vi "ENA_E5072A.vi"() -> ()   [LabVIEW 2020]
uses:
  484af209-f5fb-4e97-a5fb-2c0625b22b84.vi
  <instrlib>/Agilent ENA Series/Agilent ENA Series.lvlib
panel:
  out "종료(숨김)":bool
  out "진행상황":string
  out "저장 카운터(숨김)":i32
  out "flag(숨김)":bool
  out "진행시간":string="0d 0h 0m 0s"
  in  "자동저장":bool
  in  "작동시간(분)":i32=120 min=1
  in  "주기(분)":i32=20 min=1
  out "최종저장횟수(숨김)":string
  out "종료시간":timestamp format="%<%X\n%x>T"
  out "시작(숨김)":timestamp format="%<%X\n%x>T"
  out "실수값 [dB]":dbl
  out "주파수 [MHz]":dbl
  out "Data sheet":string[][](table)
  in  "s2p 저장":bool caption="빈 버튼"
  in  "s2p 파일명":string caption="파일명"
  in  "파일명":string
  in  "저장경로":path
  in  "이미지 저장":bool caption="빈 버튼"
  in  "Reset":bool
  in  "라디오 버튼":enum32{"Center / Span", "Start / Stop"}(radio)
  in  "Stop [MHz]":dbl
  in  "Start [MHz]":dbl
  in  "Span [MHz]":dbl=2000.0
  in  "Center [MHz]":dbl=5000.0
  in  "Value Graticule Line (0.0)":dbl format="%^.2e"
  in  "Data Format":u16(ring) items=["Logarithmic Magnitude", "Phase", "Group Delay", "Smith Chart  Linear (Lin/Phase)", "Smith Chart  Logarithmic (Log/Phase)", "Smith Chart  Complex (Real/Imag)", "Smith Chart  Impedance (R+jX)", "Smith Chart  Admittance (G+jB)", "Polar Format (Linear)", "Polar Format (Logarithmic)", "Polar Format (Re/Im)", "Linear Magnitude", "SWR", "Real", "Imaginary", "Epanded Phase", "Positive Phase"]
  in  "Measurement Parameters":u16(ring)=1 items=["S11"=0, "S21"=1, "S12"=4, "S22"=5, "A"=16, "B"=17, "R1"=20, "R2"=21, "AUX1"=24, "AUX2"=25]
  in  "VISA Resource Name":refnum<visa-resource-name>
  in  "Hold":bool=TRUE
  out "Graph":cluster{"X":dbl, "Y":dbl}[](graph)
  in  "종료":bool
  in  "데이터 읽기":bool
  in  "설정":bool
  # "PEAK"
  # ".png"
  # ".s2p"
  # "by yys"
  # "Cont"
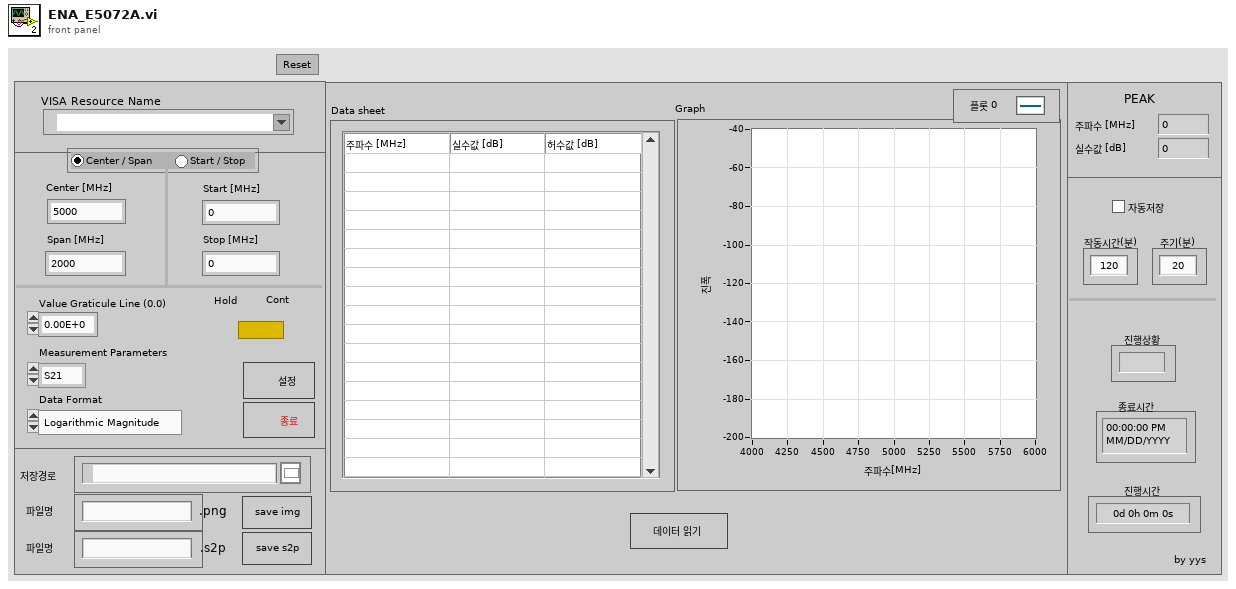
[diagram p1: front panel]
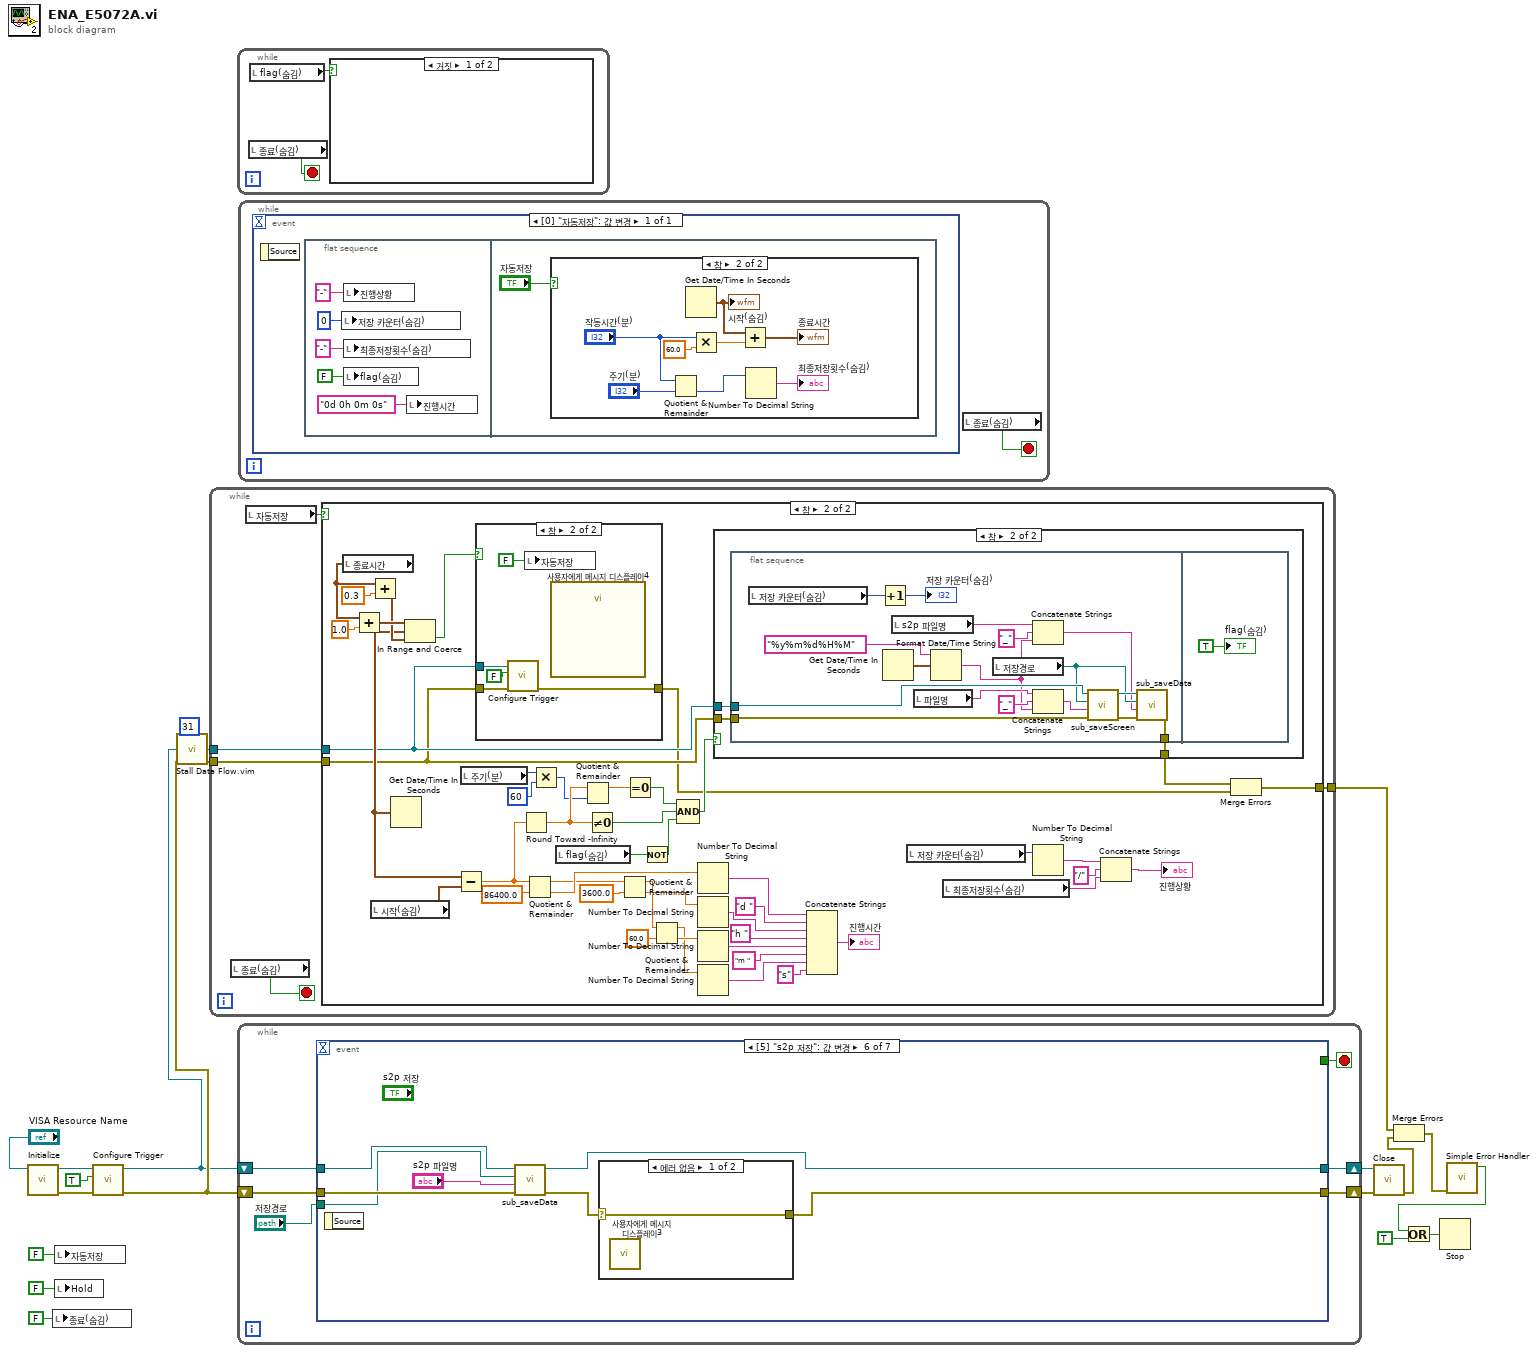
[diagram p0: block diagram]
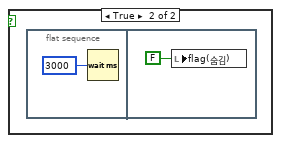
[diagram p5: hidden frame]
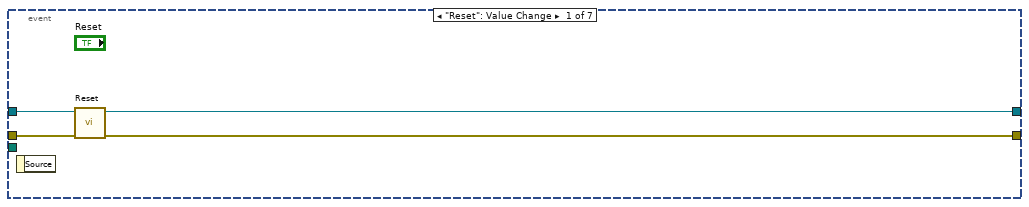
[diagram p7: hidden frame]
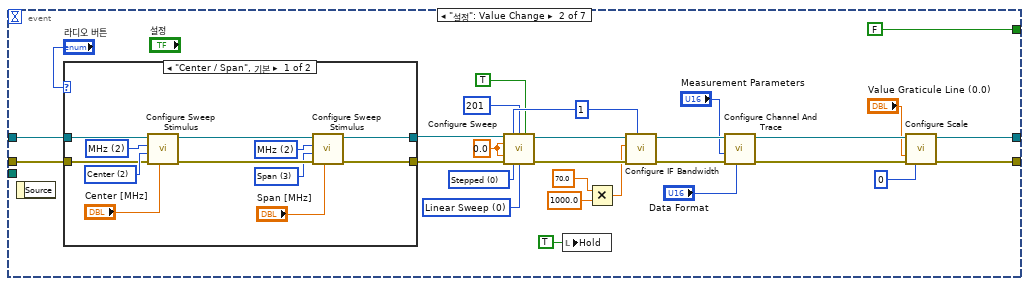
[diagram p8: hidden frame]
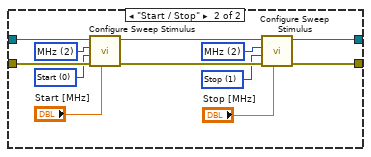
[diagram p9: hidden frame]
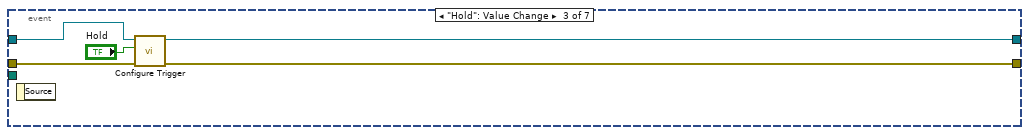
[diagram p10: hidden frame]
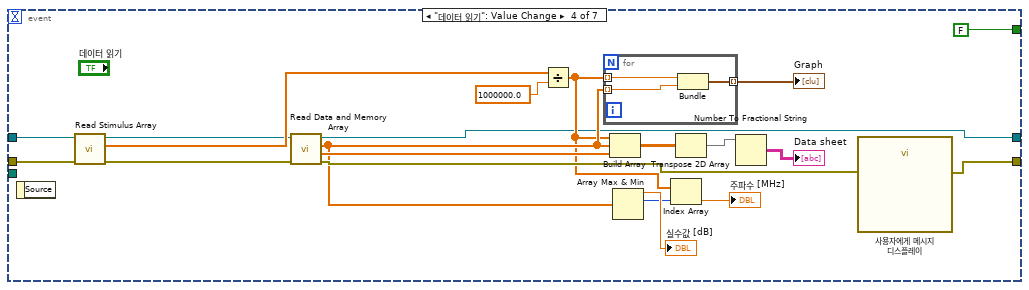
[diagram p11: hidden frame]
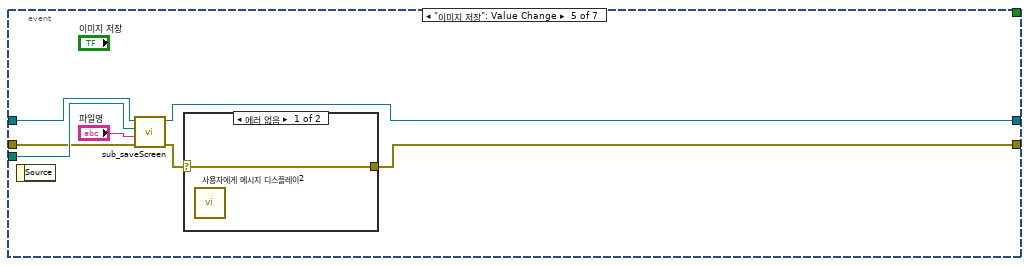
[diagram p12: hidden frame]
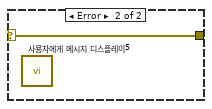
[diagram p13: hidden frame]
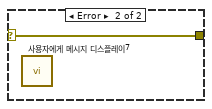
[diagram p14: hidden frame]
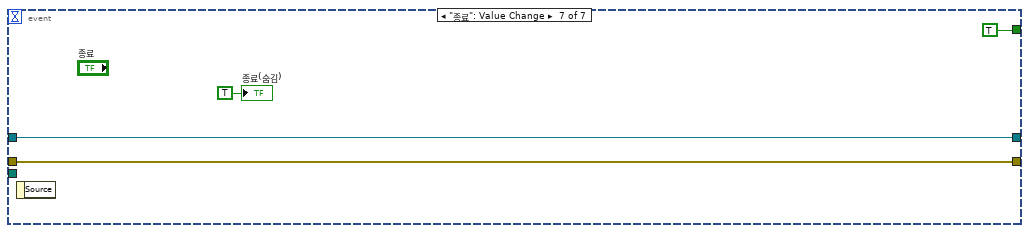
[diagram p15: hidden frame]
diagram:
  n1 = call <instrlib>:"Initialize.vi"("VISA resource name"="VISA Resource Name") -> ("error out"=w17:errorcluster, "VISA resource name out"=w18:refnum<visa-resource-name>)  [unwired: 9 in]
  n2 = local write "종료(숨김)"(FALSE ("종료(숨김)")) -> ()
  n3 = local write "자동저장"(FALSE ("자동저장")) -> ()
  n4 = local write "Hold"(FALSE ("Hold")) -> ()
  n5 = call <instrlib>:"Configure Trigger.vi"("error in (no error)"=w17, "Continuous Sweep (T: Enable)"=TRUE, "VISA resource name"=w18) -> ("error out"=w10:errorcluster, "VISA resource name out"=w9:refnum<visa-resource-name>)  [unwired: 7 in]
  n6 = call "Stall Data Flow.vim"("value in"=w9, "milliseconds to wait"=u32 31) -> ("value out"=w12:refnum<visa-resource-name>)  [unwired: 1 out]
  n7 = while {
    tunnel: w12 -> [w22]
    tunnel: w10 -> [w21]
    tunnel: [w20] -> w8
    stop <- w23 stop-if-true
    n8 = local read "종료(숨김)"() -> (w23:bool)
    n9 = local read "자동저장"() -> (w24:bool)
    n10 = case shown="참" w24 {
      tunnel: w22 -> [_ w30]
      tunnel: w21 -> [w25 w29]
      tunnel: [w25 w26] -> w20
      frame False {
      }
      frame True {
        n11 = local read "종료시간"() -> (w35:timestamp)
        n12 = Add(x=w35, y=1.0) -> (x+y=w42:timestamp)
        n13 = Add(x=w35, y=0.3) -> (x+y=w34:timestamp)
        n14 = local read "시작(숨김)"() -> (w53:timestamp)
        n15 = Get Date/Time In Seconds() -> (seconds since 1Jan1904=w31:timestamp)
        n16 = In Range and Coerce(upper limit=w42, x=w31, lower limit=w34) -> (In Range?=w44:bool)  [unwired: 1 out]
        n17 = Subtract(x=w31, y=w53) -> (x-y=w52:dbl)
        n18 = local read "주기(분)"() -> (w56:i32)
        n19 = case shown="참" w44 {
          tunnel: w30 -> [_ w76]
          tunnel: w29 -> [w73 w75]
          tunnel: [w73 w74] -> w28
          frame False {
          }
          frame True {
            n20 = call <instrlib>:"Configure Trigger.vi"("error in (no error)"=w75, "Continuous Sweep (T: Enable)"=FALSE, "VISA resource name"=w76) -> ("error out"=w74:errorcluster)  [unwired: 7 in, 1 out]
            n21 = local write "자동저장"(FALSE ("자동저장")) -> ()
            n22 = call "사용자에게 메시지 디스플레이4"() -> ()  [unwired: 10 in, 2 out]
          }
        }
        n23 = Round Toward -Infinity(1:w52) -> (0:w49:dbl)
        n24 = Quotient & Remainder(x=w52, y=86400.0) -> (x-y*floor(x/y)=w70:dbl, floor(x/y)=w72:dbl)
        n25 = Multiply(x=w56, y=60) -> (x*y=w45:i32)
        n26 = local read "flag(숨김)"() -> (w47:bool)
        n27 = Quotient & Remainder(x=w49, y=w45) -> (x-y*floor(x/y)=w54:dbl)  [unwired: 1 out]
        n28 = Not Equal To 0?(x=w49) -> (x != 0?=w50:bool)
        n29 = Quotient & Remainder(x=w70, y=3600.0) -> (x-y*floor(x/y)=w68:dbl, floor(x/y)=w71:dbl)
        n30 = Equal To 0?(x=w54) -> (x = 0?=w51:bool)
        n31 = Not(x=w47) -> (.not. x?=w46:bool)
        n32 = Quotient & Remainder(x=w68, y=60.0) -> (x-y*floor(x/y)=w67:dbl, floor(x/y)=w69:dbl)
        n33 = Compound Arithmetic op=AND ("복합 연산")(w51, w50, w46) -> (w48:bool)
        n34 = Number To Decimal String(number=w72) -> (decimal integer string=w32:string)  [unwired: 1 in]
        n35 = Number To Decimal String(number=w71) -> (decimal integer string=w66:string)  [unwired: 1 in]
        n36 = Number To Decimal String(number=w69) -> (decimal integer string=w65:string)  [unwired: 1 in]
        n37 = Number To Decimal String(number=w67) -> (decimal integer string=w64:string)  [unwired: 1 in]
        n38 = case shown="참" w48 {
          tunnel: w30 -> [_ w82]
          tunnel: w29 -> [w79 w81]
          tunnel: [w79 w80] -> w27
          frame False {
          }
          frame True {
            n39 = flat-sequence {
              tunnel: w82 -> [w98]
              tunnel: w81 -> [w86]
              tunnel: [w83] -> w80
              frame #0 {
                n40 = local read "저장 카운터(숨김)"() -> (w84:i32)
                n41 = Increment(x=w84) -> (x+1=→"저장 카운터(숨김)":i32)
                n42 = Get Date/Time In Seconds() -> (seconds since 1Jan1904=w95:timestamp)
                n43 = local read "s2p 파일명"() -> (w92:string)
                n44 = local read "파일명"() -> (w89:string)
                n45 = Format Date/Time String(time format string (%c)="%y%m%d%H%M" ("시간 포맷 문자열 (%c)"), seconds (now)=w95) -> (date/time string=w88:string)  [unwired: 1 in]
                n46 = local read "저장경로"() -> (w96:path)
                n47 = Concatenate Strings(w92, "_" ("문자열"), w88) -> (w91:string)
                n48 = Concatenate Strings(w89, "_" ("문자열"), w88) -> (w87:string)
                n49 = call "sub_saveScreen.vi"("에러 입력(에러 없음)"=w86, "파일명"=w87, "저장경로"=w96, "VISA 참조 번호 입력"=w98) -> ("에러 출력"=w85:errorcluster, "VISA 참조 번호 출력"=w97:refnum<visa-resource-name>)  [unwired: 6 in]
                n50 = call "sub_saveData.vi"("에러 입력(에러 없음)"=w85, "파일명"=w91, "저장경로"=w96, "VISA 참조 번호 입력"=w97) -> ("에러 출력"=w83:errorcluster)  [unwired: 6 in, 1 out]
              }
              frame #1 {
                "flag(숨김)" <- TRUE
              }
            }
          }
        }
        n51 = Concatenate Strings(w32, "d " ("문자열"), w66, "h " ("문자열"), w65, "m " ("문자열"), w64, "s" ("문자열")) -> (→"진행시간":string)
        n52 = local read "저장 카운터(숨김)"() -> (w39:i32)
        n53 = local read "최종저장횟수(숨김)"() -> (w33:string)
        n54 = Number To Decimal String(number=w39) -> (decimal integer string=w38:string)  [unwired: 1 in]
        n55 = Concatenate Strings(w38, "/" ("문자열"), w33) -> (→"진행상황":string)
        n56 = Merge Errors(w27, w28) -> (w26:errorcluster)
      }
    }
  }
  n57 = while {
    stop <- w101 stop-if-true
    n58 = local read "종료(숨김)"() -> (w101:bool)
    n59 = local read "flag(숨김)"() -> (w102:bool)
    n60 = case shown="거짓" w102 {
      frame False {
      }
      frame True {
        n61 = flat-sequence {
          frame #0 {
            n62 = Wait (ms)(milliseconds to wait=u32 3000 ("대기 시간 (ms)")) -> ()  [unwired: 1 out]
          }
          frame #1 {
            n63 = local write "flag(숨김)"(FALSE) -> ()
          }
        }
      }
    }
  }
  n64 = while {
    shift-right: [w110] -> w15
    shift-left: w9 -> [w106]
    shift-right: [w109] -> w14
    shift-left: w10 -> [w105]
    stop <- w107 stop-if-true
    n65 = event shown="[5] \"s2p 저장\": 값 변경" {
      selector: _ -> [_ _ _ _ _ _ _]
      dyn-events: _ -> [_ _ _ _ _ _ _]
      timeout: _ -> [_ _ _ _ _ _ _]
      tunnel: [_ FALSE _ FALSE _ _ TRUE] -> w107
      tunnel: w106 -> [w114 w118 w171 w185 w201 w210 w215]
      tunnel: w105 -> [w113 w119 w170 w183 w198 w209 w214]
      tunnel: [w112 w138 w167 w172 w197 w206 w215] -> w110
      tunnel: [w111 w137 w168 w179 w195 w204 w214] -> w109
      tunnel: "저장경로" -> [_ _ _ _ w200 w208 _]
      event "Reset": Value Change {
        n66 = event-data() -> ()  [unwired: 1 in, 1 out]
        n67 = call <instrlib>:"Reset.vi"("error in (no error)"=w113, "VISA resource name"=w114) -> ("error out"=w111:errorcluster, "VISA resource name out"=w112:refnum<visa-resource-name>)  [unwired: 8 in]
      }
      event "설정": Value Change {
        w127 = 0.0 ("Sweep Time (0.001)")
        w128 = u16 0 items=["Linear Sweep", "Logarithmic Sweep", "Segment Sweep", "Power Sweep", "DC Bias"] ("Sweep Type (0: Linear Sweep)")
        w129 = u16 0 items=["Stepped", "Swept", "Fast Stepped Mode", "Fast Swept Mode"] ("Sweep Mode (0: Stepped)")
        w134 = 1 ("Channel (1)")
        n68 = event-data() -> ()  [unwired: 1 in, 1 out]
        n69 = case shown="\"Center / Span\", 기본" "라디오 버튼" {
          tunnel: [w146 w156] -> w117
          tunnel: [w147 w155] -> w116
          tunnel: w119 -> [w144 w160]
          tunnel: w118 -> [w145 w157]
          frame "Center / Span", Default {
            w151 = u16 2 items=["Hz", "kHz", "MHz", "GHz", "dBm", "s", "V"] ("Unit (0: Hz)")
            w149 = u16 2 items=["Hz", "kHz", "MHz", "GHz", "dBm", "s", "V"] ("Unit (0: Hz)")
            w152 = u16 3 items=["Start", "Stop", "Center", "Span"] ("Stimulus (0: Start)")
            w150 = u16 2 items=["Start", "Stop", "Center", "Span"] ("Stimulus (0: Start)")
            n70 = call <instrlib>:"Configure Sweep Stimulus.vi"("Parameter (0.0)"="Center [MHz]", "error in (no error)"=w144, "Stimulus (0: Start)"=w150, "Unit (0: Hz)"=w149, "VISA resource name"=w145) -> ("error out"=w153:errorcluster, "VISA resource name out"=w143:refnum<visa-resource-name>)  [unwired: 5 in]
            n71 = call <instrlib>:"Configure Sweep Stimulus.vi"("Parameter (0.0)"="Span [MHz]", "error in (no error)"=w153, "Stimulus (0: Start)"=w152, "Unit (0: Hz)"=w151, "VISA resource name"=w143) -> ("error out"=w146:errorcluster, "VISA resource name out"=w147:refnum<visa-resource-name>)  [unwired: 5 in]
          }
          frame "Start / Stop" {
            w161 = u16 2 items=["Hz", "kHz", "MHz", "GHz", "dBm", "s", "V"] ("Unit (0: Hz)")
            w162 = u16 1 items=["Start", "Stop", "Center", "Span"] ("Stimulus (0: Start)")
            w159 = u16 0 items=["Start", "Stop", "Center", "Span"] ("Stimulus (0: Start)")
            w158 = u16 2 items=["Hz", "kHz", "MHz", "GHz", "dBm", "s", "V"] ("Unit (0: Hz)")
            n72 = call <instrlib>:"Configure Sweep Stimulus.vi"("Parameter (0.0)"="Start [MHz]", "error in (no error)"=w160, "Stimulus (0: Start)"=w159, "Unit (0: Hz)"=w158, "VISA resource name"=w157) -> ("error out"=w165:errorcluster, "VISA resource name out"=w163:refnum<visa-resource-name>)  [unwired: 5 in]
            n73 = call <instrlib>:"Configure Sweep Stimulus.vi"("Parameter (0.0)"="Stop [MHz]", "error in (no error)"=w165, "Stimulus (0: Start)"=w162, "Unit (0: Hz)"=w161, "VISA resource name"=w163) -> ("error out"=w156:errorcluster, "VISA resource name out"=w155:refnum<visa-resource-name>)  [unwired: 5 in]
          }
        }
        n74 = call <instrlib>:"Configure Sweep.vi"("VISA resource name"=w116, "Channel (1)"=w134, "Number of Measurement Points (201)"=201, "Auto Sweep Time (F: Off)"=TRUE, "Sweep Time (0.001)"=w127, "Delay Time (0.001)"=w127, "error in (no error)"=w117, "Sweep Mode (0: Stepped)"=w129, "Sweep Type (0: Linear Sweep)"=w128) -> ("VISA resource name out"=w136:refnum<visa-resource-name>, "error out"=w135:errorcluster)  [unwired: 5 in]
        n75 = local write "Hold"(TRUE ("Hold")) -> ()
        n76 = Multiply(x=70.0, y=1000.0) -> (x*y=w132:dbl)
        n77 = call <instrlib>:"Configure IF Bandwidth.vi"("Channel (1)"=w134, "error in (no error)"=w135, "IF Bandwidth (100000.0)"=w132, "VISA resource name"=w136) -> ("error out"=w124:errorcluster, "VISA resource name out"=w125:refnum<visa-resource-name>)  [unwired: 6 in]
        n78 = call <instrlib>:"Configure Channel And Trace.vi"("Data Format (0: Logarithmic Magnitude)"="Data Format", "error in (no error)"=w124, "Measurement Parameters (0: S11)"="Measurement Parameters", "VISA resource name"=w125) -> ("error out"=w141:errorcluster, "VISA resource name out"=w142:refnum<visa-resource-name>)  [unwired: 6 in]
        n79 = call <instrlib>:"Configure Scale.vi"("VISA resource name"=w142, "Value Graticule Line (0.0)"="Value Graticule Line (0.0)", "error in (no error)"=w141, "Reference Graticule Line (5)"=0) -> ("VISA resource name out"=w138:refnum<visa-resource-name>, "error out"=w137:errorcluster)  [unwired: 10 in]
      }
      event "Hold": Value Change {
        n80 = event-data() -> ()  [unwired: 1 in, 1 out]
        n81 = call <instrlib>:"Configure Trigger.vi"("error in (no error)"=w170, "Continuous Sweep (T: Enable)"="Hold", "VISA resource name"=w171) -> ("error out"=w168:errorcluster, "VISA resource name out"=w167:refnum<visa-resource-name>)  [unwired: 7 in]
      }
      event "데이터 읽기": Value Change {
        n82 = event-data() -> ()  [unwired: 1 in, 1 out]
        n83 = call <instrlib>:"Read Stimulus Array.vi"("error in (no error)"=w183, "VISA resource name"=w185) -> ("error out"=w182:errorcluster, "Stimulus Data"=w190:dbl[], "VISA resource name out"=w184:refnum<visa-resource-name>)  [unwired: 7 in]
        n84 = call <instrlib>:"Read Data and Memory Array.vi"("error in (no error)"=w182, "VISA resource name"=w184) -> ("error out"=w180:errorcluster, "Secondary / Imaginary"=w188:dbl[], "Primary / Real"=w177:dbl[], "VISA resource name out"=w172:refnum<visa-resource-name>)  [unwired: 6 in]
        n85 = Divide(x=w190, y=1000000.0) -> (x/y=w174:dbl[])
        n86 = for {
          tunnel: w174 -> [w194] mode=indexing
          tunnel: w177 -> [w193] mode=indexing
          tunnel: [w192] -> w181 mode=indexing
          n87 = Bundle(w194, w193) -> (w192:cluster{dbl, dbl})  [unwired: 1 in]
        }
        "Graph" <- w181
        n88 = Build Array(w174, w177, w188) -> (w187:dbl[][])
        n89 = Array Max & Min(array=w177) -> (max value=→"실수값 [dB]":dbl, max index (indices)=w175:i32)  [unwired: 2 out]
        n90 = Index Array(array=w174, index=w175) -> (element=→"주파수 [MHz]":dbl)
        n91 = Transpose 2D Array(2D array=w187) -> (transposed array=w186:dbl[][])
        n92 = Number To Fractional String(number=w186) -> (F-format string=→"Data sheet":string[][])  [unwired: 3 in]
        n93 = call "사용자에게 메시지 디스플레이"("error in (no error)"=w180) -> ("error out"=w179:errorcluster)  [unwired: 9 in, 1 out]
      }
      event "이미지 저장": Value Change {
        n94 = event-data() -> ()  [unwired: 1 in, 1 out]
        n95 = call "sub_saveScreen.vi"("에러 입력(에러 없음)"=w198, "파일명"="파일명", "저장경로"=w200, "VISA 참조 번호 입력"=w201) -> ("에러 출력"=w196:errorcluster, "VISA 참조 번호 출력"=w197:refnum<visa-resource-name>)  [unwired: 6 in]
        n96 = case shown="에러 없음" w196 {
          selector: w196 -> [w202 w203]
          tunnel: [w202 w203] -> w195
          frame No Error {
            n97 = call "사용자에게 메시지 디스플레이2"() -> ()  [unwired: 10 in, 2 out]
          }
          frame Error {
            n98 = call "사용자에게 메시지 디스플레이5"() -> ()  [unwired: 10 in, 2 out]
          }
        }
      }
      event "s2p 저장": Value Change {
        n99 = event-data() -> ()  [unwired: 1 in, 1 out]
        n100 = call "sub_saveData.vi"("에러 입력(에러 없음)"=w209, "파일명"="s2p 파일명", "저장경로"=w208, "VISA 참조 번호 입력"=w210) -> ("에러 출력"=w205:errorcluster, "VISA 참조 번호 출력"=w206:refnum<visa-resource-name>)  [unwired: 6 in]
        n101 = case shown="에러 없음" w205 {
          selector: w205 -> [w211 w212]
          tunnel: [w211 w212] -> w204
          frame No Error {
            n102 = call "사용자에게 메시지 디스플레이3"() -> ()  [unwired: 10 in, 2 out]
          }
          frame Error {
            n103 = call "사용자에게 메시지 디스플레이7"() -> ()  [unwired: 10 in, 2 out]
          }
        }
      }
      event "종료": Value Change {
        n104 = event-data() -> ()  [unwired: 1 in, 1 out]
        "종료(숨김)" <- TRUE ("종료 2")
      }
    }
  }
  n105 = while {
    stop <- w217 stop-if-true
    n106 = event shown="[0] \"자동저장\": 값 변경" {
      selector: _ -> [_]
      dyn-events: _ -> [_]
      timeout: _ -> [_]
      event "자동저장": Value Change {
        n107 = event-data() -> ()  [unwired: 1 in, 1 out]
        n108 = flat-sequence {
          frame #0 {
            n109 = local write "저장 카운터(숨김)"(0 ("숫자형")) -> ()
            n110 = local write "진행상황"("-" ("진행상황")) -> ()
            n111 = local write "최종저장횟수(숨김)"("-" ("진행상황")) -> ()
            n112 = local write "flag(숨김)"(FALSE) -> ()
            n113 = local write "진행시간"("0d 0h 0m 0s" ("진행시간")) -> ()
          }
          frame #1 {
            n114 = case shown="참" "자동저장" {
              frame False {
              }
              frame True {
                n115 = Quotient & Remainder(x="작동시간(분)", y="주기(분)") -> (floor(x/y)=w225:i32)  [unwired: 1 out]
                n116 = Get Date/Time In Seconds() -> (seconds since 1Jan1904=w226:timestamp)
                "시작(숨김)" <- w226
                n117 = Multiply(x="작동시간(분)", y=60.0) -> (x*y=w230:dbl)
                n118 = Add(x=w226, y=w230) -> (x+y=→"종료시간":timestamp)
                n119 = Number To Decimal String(number=w225) -> (decimal integer string=→"최종저장횟수(숨김)":string)  [unwired: 1 in]
              }
            }
          }
        }
      }
    }
    n120 = local read "종료(숨김)"() -> (w217:bool)
  }
  n121 = call <instrlib>:"Close.vi"("error in (no error)"=w14, "VISA resource name"=w15) -> ("error out"=w6:errorcluster)  [unwired: 9 in]
  n122 = Merge Errors(w8, w6) -> (w7:errorcluster)
  n123 = call <vilib>:"Simple Error Handler.vi"("error in (no error)"=w7) -> ("error?"=w1:bool)  [unwired: 4 in, 4 out]
  n124 = Or(x=w1, y=TRUE) -> (x .or. y?=w2:bool)
  n125 = Stop(stop? (T)=w2) -> ()
